vi "DDS Channel to CS Pin.vi"(1 "channel number (1)":u8=1 min=1 max=4 step=1) -> (0 "CS pin":T1)   [LabVIEW 2013]
doc: "Given a channel number, returns the enum representing the channel's CS pin."
uses:
  DDS CS pins.ctl
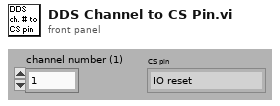
[diagram p1: front panel]
types:
  T1 = typedef "DDS CS pins.ctl" = enum8{"IO reset", "Ch. 4 CS", "Ch. 3 CS", "Ch. 2 CS", "Ch. 1 CS"}
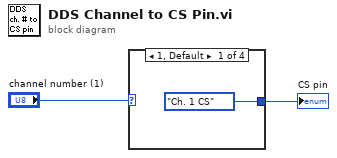
[diagram p0: block diagram]
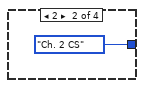
[diagram p2: hidden frame]
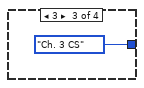
[diagram p3: hidden frame]
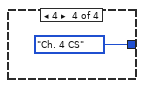
[diagram p4: hidden frame]
diagram:
  n1 = case shown="1, Default" "channel number (1)" {
    tunnel: [DDS_CS_pins."Ch. 1 CS" ("DDS CS pins") DDS_CS_pins."Ch. 2 CS" ("DDS CS pins") DDS_CS_pins."Ch. 3 CS" ("DDS CS pins") DDS_CS_pins."Ch. 4 CS" ("DDS CS pins")] -> w1
    frame 1, Default {
    }
    frame 2 {
    }
    frame 3 {
    }
    frame 4 {
    }
  }
  "CS pin" <- w1
